vi "Data Type Registration Example.vi"() -> ()   [LabVIEW 2016, in "Stream Mediator.lvlib"]
uses:
  <userlib>/Composed Systems/Stream/Mediator/Stream Mediator.lvlib
  <vilib>/Composed Systems/Stream/Mediator/Classes/Message Double/Message Double.lvclass
  <vilib>/Composed Systems/Stream/Mediator/Classes/Message Transport Queue/Message Transport Queue.lvclass
  <vilib>/Composed Systems/Stream/Mediator/Classes/Message Transport Event/Message Transport Event.lvclass
  <userlib>/Composed Systems/Stream/Mediator/Classes/Message Broker Interface Ref/Message Broker Interface Ref.lvclass
  C:/Program Files (x86)/National Instruments/LabVIEW 2016/user.lib/Composed Systems/Stream/Mediator/Classes/Message Broker Interface/Message Broker Interface.lvclass
panel:
  out "Value":dbl
  in  "Data":dbl
  in  "Publish Rate":u32=100
  in  "Stop":bool
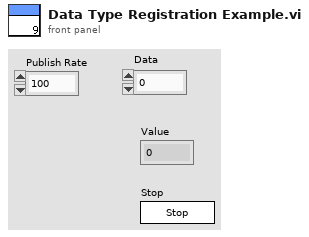
[diagram p1: front panel]
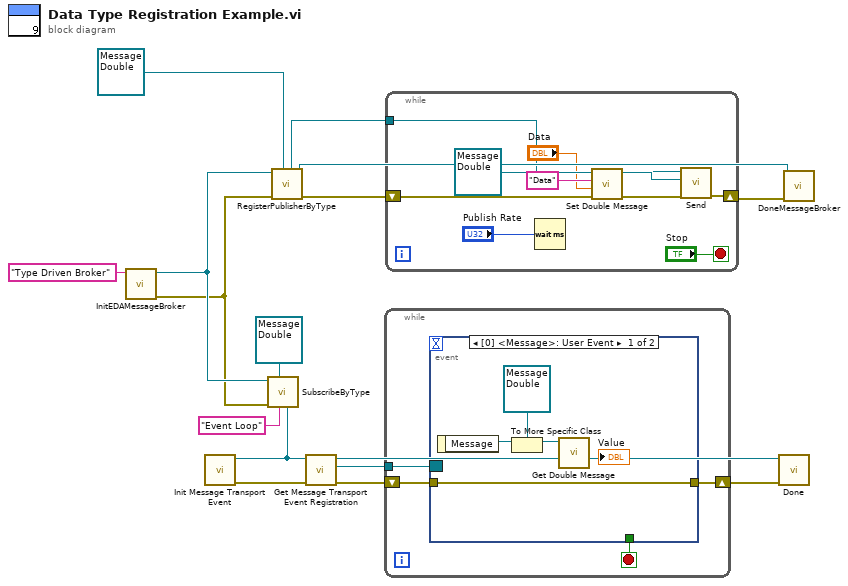
[diagram p0: block diagram]
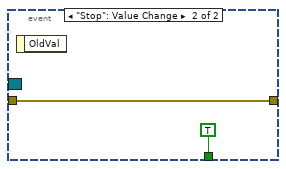
[diagram p2: hidden frame]
diagram:
  n1 = call <vilib>:"InitEDAMessageBroker.vi"("Broker Name"="Type Driven Broker") -> ("error out"=w12:errorcluster, "EDA Message Broker Interface Ref out"=w13:refnum<class "EDA Message Broker Interface Ref.lvclass">)  [unwired: 9 in]
  n2 = call <vilib>:"Init Message Transport Event.vi"() -> ("error out"=w10:errorcluster, "Message Transport Event out"=w9:refnum<class "Message Transport Event.lvclass">)  [unwired: 10 in]
  n3 = call <vilib>:"SubscribeByType.vi"("Message Transport Interface"=w9, "Subscriber Name"="Event Loop", "Event"=refnum<class "Message Double.lvclass"> refnum ("Stream Mediator.lvlib:Message Double.lvclass"), "error in (no error)"=w12, "Message Broker Interface in"=w13) -> ()  [unwired: 5 in, 2 out]
  n4 = call <vilib>:"RegisterPublisherByType.vi"("Event"=refnum<class "Message Double.lvclass"> refnum ("Stream Mediator.lvlib:Message Double.lvclass"), "error in (no error)"=w12, "EDA Message Broker Interface Ref in"=w13) -> ("error out"=w14:errorcluster, "EDA Message Broker Interface Ref out"=w3:refnum<class "EDA Message Broker Interface Ref.lvclass">, "Transport"=w15:refnum<class "Message Transport Queue.lvclass">)  [unwired: 5 in, 1 out]
  n5 = call <vilib>:"Get Message Transport Event Registration.vi"("error in (no error)"=w10, "Message Transport Event in"=w9) -> ("error out"=w7:errorcluster, "Event Registration Refnum"=w8:refnum<event-registration>, "Message Transport Event out"=w5:refnum<class "Message Transport Event.lvclass">)  [unwired: 6 in, 1 out]
  n6 = while {
    tunnel: w8 -> [w20]
    shift-right: [w18] -> w6
    shift-left: w7 -> [w19]
    stop <- w17 stop-if-true
    n7 = event shown="[0] <Message>: User Event" {
      selector: w20 -> [_ _]
      dyn-events: _ -> [_ _]
      timeout: _ -> [_ _]
      tunnel: w19 -> [w25 w26]
      tunnel: [w25 w26] -> w18
      tunnel: [_ TRUE] -> w17
      event User Event {
        n8 = event-data() -> ("Message"=w23:refnum<class "Message Interface.lvclass">)  [unwired: 1 in]
        n9 = To More Specific Class(target class=refnum<class "Message Double.lvclass"> refnum ("Stream Mediator.lvlib:Message Double.lvclass"), reference=w23) -> (specific class reference=w22:refnum<class "Message Double.lvclass">)  [unwired: 1 in, 1 out]
        n10 = call <vilib>:"Get Double Message.vi"("Message Double in"=w22) -> ("Value"=→"Value":dbl)  [unwired: 7 in, 3 out]
      }
      event "Stop": Value Change {
        n11 = event-data() -> ()  [unwired: 1 in, 1 out]
      }
    }
  }
  n12 = while {
    tunnel: w15 -> [w30]
    shift-right: [w28] -> w4
    shift-left: w14 -> [w31]
    stop <- "Stop" stop-if-true
    n13 = Wait (ms)(milliseconds to wait="Publish Rate") -> ()  [unwired: 1 out]
    n14 = call <vilib>:"Set Double Message.vi"("error in (no error)"=w31, "Value"="Data", "Name"="Data", "Message Double in"=refnum<class "Message Double.lvclass"> refnum ("Message Double.lvclass")) -> ("error out"=w29:errorcluster, "Message Double out"=w32:refnum<class "Message Double.lvclass">)  [unwired: 6 in]
    n15 = call-dynamic "Send.vi"("error in (no error)"=w29, "Message"=w32, "Message Transport Queue in"=w30) -> ("error out"=w28:errorcluster)  [unwired: 6 in, 2 out]
  }
  n16 = call-dynamic "Done.vi"("error in (no error)"=w6, "Message Transport Event in"=w5) -> ()  [unwired: 8 in, 2 out]
  n17 = call <userlib>:"DoneMessageBroker.vi"("error in (no error)"=w4, "Message Broker Interface Ref in"=w3) -> ()  [unwired: 8 in, 2 out]
